vi "Read Image File Directory.vi"(3 "Litt/BigEnd":bool, 4 "Im_File_Dir Offs":i32, 5 "Image Data in":u8[](array[numeric])) -> (1 "Directories":cluster{"Tags":T1[]}[](array[cluster]), 2 "Image Data out":u8[](array[numeric]))   [LabVIEW 2015, in "Tiff reader.lvlib"]
doc: "Reads the tags and associated data in a tiff file byte stream (Image Data in) starting at an offset (Image File Directory Offset) which is determined using the Read Header.vi. Returns an array of clusters containing the tag and location and format of the assocaited data."
uses:
  Tiff reader.lvlib
  IFD Entry.ctl
  FieldTypes.ctl
panel:
  out "size(s)":i32
  out "Array":u32[](array[numeric])
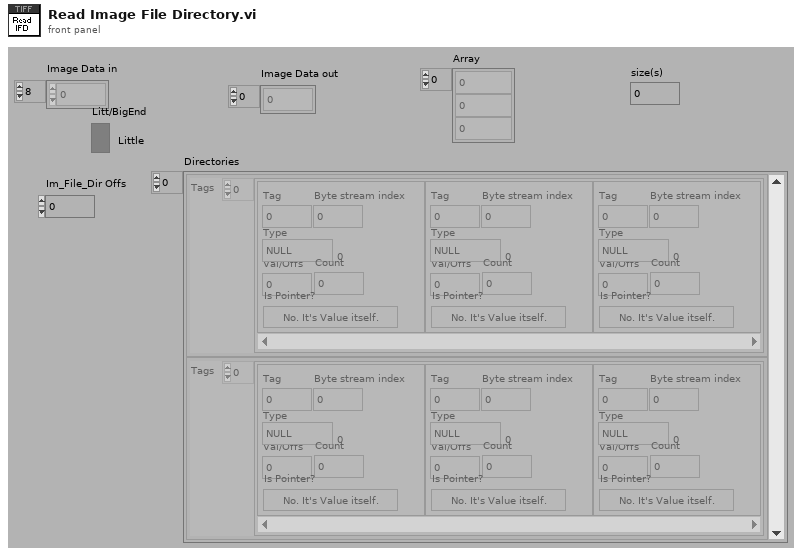
[diagram p1: front panel]
types:
  T1 = typedef "Tiff reader.lvlib/IFD Entry.ctl" = cluster{"Tag":u16, "Type":T2, "Count":u32, "Val/Offs":u32, "Is Pointer?":bool, "Byte stream index":i32}
  T2 = typedef "Tiff reader.lvlib/FieldTypes.ctl" = enum16{"NULL", "U8", "ASCII7", "U16", "U32", "RATIONAL", "SByte(I8)", "Undef(8Bit)", "I16", "I32", "SRat(4B:4B)", "SGL(4Byte)", "DBL(8Byte)"}
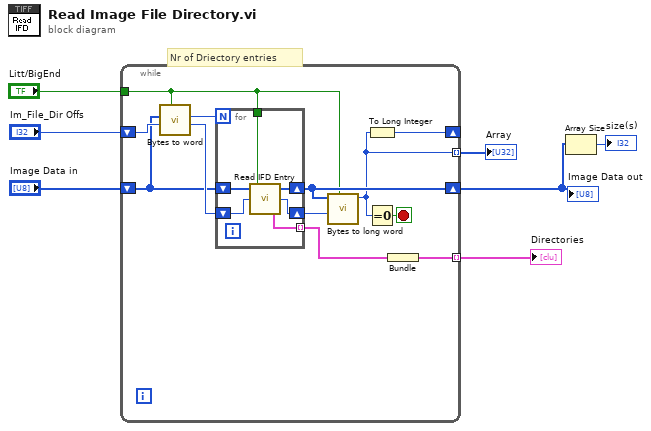
[diagram p0: block diagram]
diagram:
  # "Nr of Driectory entries"
  n1 = while {
    shift-right: [w14] -> _
    shift-left: "Im_File_Dir Offs" -> [w19]
    tunnel: "Litt/BigEnd" -> [w11]
    tunnel: [w10] -> w5 mode=indexing
    shift-right: [w17] -> w2
    shift-left: "Image Data in" -> [w13]
    tunnel: [w8] -> w1 mode=indexing
    stop <- w15 stop-if-true
    n2 = call "Bytes to word.vi"("Litt/BigEnd"=w11, "Index"=w19, "Image Data in"=w13) -> ("Index+2"=w18:i32, "Word"=w12:u16)  [unwired: 1 in, 4 out]
    n3 = for {
      N: w12 -> [_]
      shift-right: [w23] -> w17
      shift-left: w13 -> [w24]
      shift-right: [w22] -> w16
      shift-left: w18 -> [w25]
      tunnel: [w21] -> w9 mode=indexing
      tunnel: w11 -> [w20]
      n4 = call "Read IFD Entry.vi"("Litt/BigEnd"=w20, "Directory Offset in"=w25, "Image Data in"=w24) -> ("Cluster"=w21:T1, "Next Directory Offset Out\n(IN + 12)"=w22:i32, "Image Data Out"=w23:u8[])
    }
    n5 = call "Bytes to long word.vi"("Litt/BigEnd"=w11, "Index"=w16, "Image Data in"=w17) -> ("U32"=w10:u32)  [unwired: 6 out]
    n6 = To Long Integer(number=w10) -> (32bit integer=w14:i32)
    n7 = Equal To 0?(x=w10) -> (x = 0?=w15:bool)
    n8 = Bundle(w9) -> (w8:cluster{T1[]})  [unwired: 1 in]
  }
  "Image Data out" <- w2
  "Directories" <- w1
  "Array" <- w5
  n9 = Array Size(array=w2) -> (size(s)=→"size(s)":i32)
